vi "AlliGator Get Optimal IRF from Decay v2.vi"(8 "error in (no error)":errorcluster, 11 "Selected Plot Info":T2={"Multiplot XY Graph"=refnum, "Mouse Coordinates"={"Horizontal"=0, "Vertical"=0}, "Plot Index"=-1}) -> (0 "Error Out":errorcluster, 2 "Message":string, 3 "Extracted IRF":cluster{"t Array":dbl[], "IRF Array":dbl[]})   [LabVIEW 2021, in "AlliGator IRF.lvlib"]
doc: "Extract IRF from single-exponential decay by deconvolution and optimization of the time constant."
uses:
  AlliGator IRF.lvlib
  Graphs/XY Graph/XY Graph Selected Plot Info.ctl
  Graphs/XY Graph/XY Graph Refnum.ctl
  <vilib>/Utility/miscctls.llb/LVPoint32TypeDef.ctl
  Settings/AlliGator Settings List.ctl
  AlliGator IRF Optimization Controls.ctl
  AlliGator IRF Deconvolution Metrics.ctl
  Fits/IRF(X)PSED/IRF(X)PSED Fixed Parameters v3.ctl
  Fits/IRF(X)PSED/IRF(X)PSED Extraction Options.ctl
  Fits/IRF(X)PSED/Fourier Series Smoothing Option.ctl
  Fits/IRF(X)PSED/Fourier Series Truncation.ctl
  Fits/IRF(X)PSED/IRF Extraction Method.ctl
  Fits/IRF(X)PSED/Decay Fit Options v4.ctl
  Fits/Decay Convolution/Decay Model.ctl
  Fits/Residual Type.ctl
  Fits/IRF(X)PSED/Fit Weights Type v2.ctl
  Fits/Non-linear Fitting Method v2.ctl
  Fits/Fit Calculation Method.ctl
  Fits/Non-linear Fitting Algorithm.ctl
  Variant/Variant to Data/Variant to I32.vi
  Graphs/XY Graph/XY Graph Add Single Plot with Name.vi
  Graphs/XY Graph/XY Graph Add-Ons.lvlib
  Settings/AlliGator Settings.lvlib
  Notebook/Notebook.lvlib
  Fits/Fits.lvlib
  Variant/Variant to Data/Variant to Data.lvlib
panel:
  in  "Tab Control":T1(tab)
  out "Optimization Graph":cluster{"X Array":dbl[], "Y Array":dbl[]}[](graph)
  out "Power Spectrum Graph":dbl[][](graph)
  in  "Plot Names":string[](array[string])=["Tail Average", "Tail Average SG", "Tail SDV", "Tail SDV S-G", "Tail Max", "Tail Max S-G", "Tail SDV x Average", "Tail SDV x Average S-G", "Slope", "Slope S-G", "Residuals ACF SDV", "Residuals ACF SDV S-G", "Delta tau", "Delta tau S-G"]
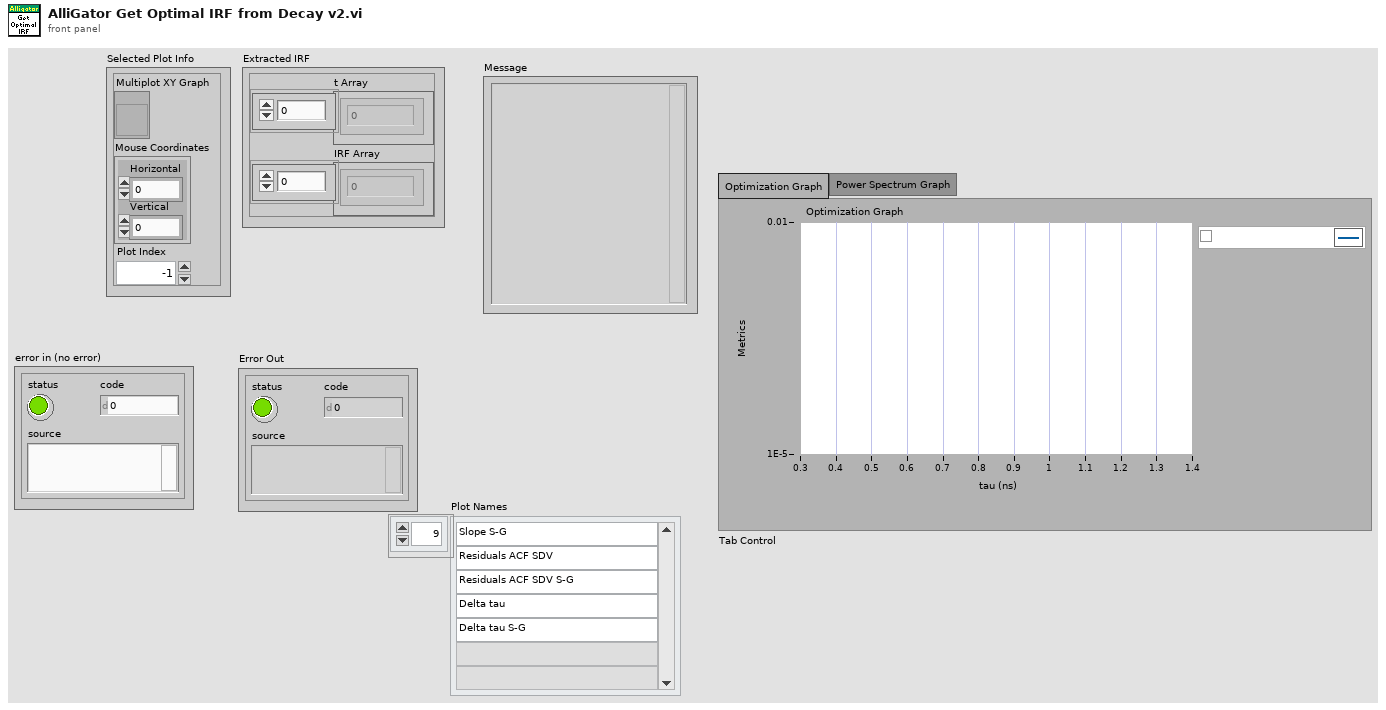
[diagram p1: front panel]
types:
  T1 = enum32{"Optimization Graph", "Power Spectrum Graph"}
  T2 = typedef "XY Graph Add-Ons.lvlib/XY Graph Selected Plot Info.ctl" = cluster{"Multiplot XY Graph":T3, "Mouse Coordinates":T4, "Plot Index":i32}
  T3 = typedef "XY Graph Add-Ons.lvlib/XY Graph Refnum.ctl" = refnum<vi>
  T4 = typedef "LVPoint32TypeDef.ctl" = cluster{"Horizontal":i32, "Vertical":i32}
  T5 = typedef "Fits.lvlib/IRF(X)PSED Extraction Options.ctl" = cluster{"Time Constant for IRF Extraction":dbl[unit], "IRF Order":i32, "Fourier Series Smoothing":T6, "Noise Threshold":dbl, "Smoothing Width":dbl, "Fourier Series Truncation":T7, "Truncation Order":i32, "Save Power Spectrum":bool, "Smoothing":bool, "Smoothing Parameter":dbl, "Smoothing Order":u32, "Method":T8}
  T6 = typedef "Fits.lvlib/Fourier Series Smoothing Option.ctl" = enum16{"None", "Lanczos Factors", "Fejer Summation"}
  T7 = typedef "Fits.lvlib/Fourier Series Truncation.ctl" = enum16{"Automatic", "Fixed"}
  T8 = typedef "Fits.lvlib/IRF Extraction Method.ctl" = enum16{"Direct", "Topless", "Toeplitz"}
  T9 = typedef "Fits.lvlib/IRF(X)PSED Fixed Parameters v3.ctl" = cluster{"order":i32, "T":dbl, "Time Constant Array":dbl[], "{S_k, C_k, phi_k, e_k} arrays":cluster{"S_k Array":dbl[], "C_k Array":dbl[], "phi_k Array":dbl[], "e_k Array":dbl[]}, "IRF Extraction Options":T5}
  T10 = typedef "AlliGator Settings.lvlib/AlliGator Settings List.ctl" = enum16{"GUI:Visible Settings Tab", "GUI:Last Run Version", "Source Image:Use Image Histogram for Contrast", "Source Image:Low Count Pixels Rejection Options", "Source Image:High Count Pixels Rejection Options", "Source Image:Use Image Brightness", "Source Image:Blend Overlay with Image Background", "Source Image:Use Fixed ROI Diameter", "Source Image:ROI Diameter", "Source Image:ROI Center Color", "Source Image:Peak Threshold", "Source Image:Intensity Threshold", "Source Image:Image Binning Options", "Source Image:Image Smoothing Options", "Source Image:Image Histogram Active", "Source Image:Invert Binary Mask", "Source Image:Hot Pixel Removal", "Source Image:Overlay Analyzed ROI Center", "Source Image:Auto-Adjust Contrast", "Source Image:Histogram Lower Percentile", "Source Image:Histogram Upper Percentile", "Source Image:Save Source Image", "Source Image:Scale Bar Options", "Source Image:Image Resolution (Pixel Size)", "Source Image:Flatfield Correction", "Source Image:Show Dead Left Columns Correction", "Source Image:Dead Left Columns Correction", "Source Image:Image Pre-Processing Operations Order", "Source Image:Overlay ROI Median", "Source Image:Median Overlay Color", "Data Information:Gate Width", "Data Information:Nanotime Gate Separation", "Data Information:Macrotime Gate Separation", "Data Information:Gate Step", "Data Information:# Gates", "Data Information:Gate Image Exposure", "Data Information:Gate Image Integration", "Data Information:Gates to Skip", "Data Information:Gates to Keep", "Data Information:Define Gates to", "Data Information:Channel Name", "Data Information:Available Channel Names", "Data Information:Channel Arithmetic", "Data Information:Background File Subtraction", "Data Information:Background File", "Data Information:Background Scaling Factor", "Data Information:Background Pile-up Correction", "Data Information:Background Pixel Well Capacity", "Data Information:Laser Period", "Data Information:SYNC Period", "Data Information:Pile-up Correction", "Data Information:Pixel Well Capacity", "Data Information:Dataset Scaling Factor", "Fluorescence Decay_Decay Pre-Processing:Reverse Gates", "Fluorescence Decay_Decay Pre-Processing:Verbose Decay Pre-Processing", "Fluorescence Decay_Decay Pre-Processing:Use Decay Pre-Processing", "Fluorescence Decay_Decay Pre-Processing:Background Subtraction", "Fluorescence Decay_Decay Pre-Processing:Background Definition Range", "Fluorescence Decay_Decay Pre-Processing:Baseline Subtraction Method", "Fluorescence Decay_Decay Pre-Processing:Decay Pre-Processing Operations Order", "Fluorescence Decay_Decay Pre-Processing:Smoothing Parameter", "Fluorescence Decay_Decay Pre-Processing:Shift Decay", "Fluorescence Decay_Decay Pre-Processing:Decay Shift Parameters", "Fluorescence Decay_Decay Pre-Processing:Fold Decay", "Fluorescence Decay_Decay Pre-Processing:# Folds", "Fluorescence Decay_Decay Pre-Processing:1-Normalize Decay", "Fluorescence Decay_Decay Pre-Processing:[0-1]-Normalize Decay", "Fluorescence Decay_Decay Pre-Processing:Smoothen Decay", "Fluorescence Decay_Decay Pre-Processing:Extrapolate Decay", "Fluorescence Decay_Decay Pre-Processing:Use Periodicity", "Fluorescence Decay_Decay Pre-Processing:Use Cursors", "Fluorescence Decay_Decay Pre-Processing:Tail Fraction", "Fluorescence Decay_Decay Pre-Processing:Head Fraction", "Fluorescence Decay_Decay Pre-Processing:Additional Points", "Fluorescence Decay_Decay Pre-Processing:Straighten Decay", "Fluorescence Decay_Decay Pre-Processing:Constant Background", "Fluorescence Decay_Decay Pre-Processing:Pixel-Normalize Decay", "Fluorescence Decay_Advanced Analysis:Extract IRF instead of Decay", "Fluorescence Decay_Advanced Analysis:IRF Extraction Options", "Fluorescence Decay_Advanced Analysis:IRF Optimization Options", "Fluorescence Decay_Advanced Analysis:Square Pulse Options", "Fluorescence Decay_Advanced Analysis:IRF Order", "Fluorescence Decay_Advanced Analysis:IRF Time Constants", "Fluorescence Decay_Advanced Analysis:Wavelet Analysis Options", "Fluorescence Decay_Advanced Analysis:Average Lifetime Options", "Fluorescence Decay_Fit Options:Fit Options", "Fluorescence Decay_Fit Options:Use Legacy Fitting Approach", "Fluorescence Decay_Fit Options:Use Data Information Laser Period", "Fluorescence Decay_Fit Parameters:Displayed Fit Parameters", "Fluorescence Decay_Fit Parameters:Fit Parameter Constraints", "Fluorescence Decay_Fit Parameters:Export Tabulated Results", "Fluorescence Decay_Fit Parameters:MLE Baseline Offset Type", "Fluorescence Decay_Fit Parameters:MLE Baseline Offset", "Fluorescence Decay_Fit Parameters:Guess Parameter Names", "Fluorescence Decay_Fit Parameters:Guess Parameter Values", "Fluorescence Decay_Fit Parameters:Guess Parameters Options", "Fluorescence Decay_Fit Parameters:Optimal Offset Selection Criterion", "Fluorescence Decay_Styles:Show Last Decay Only", "Fluorescence Decay_Styles:Decay Graph Color Array", "Fluorescence Decay:Decay Graph Active", "Fluorescence Decay Statistics:Min Peak Value", "Fluorescence Decay Statistics:Reject Low Decay Peak Pixels", "Fluorescence Decay Statistics:Reject High Decay Peak Pixels", "Fluorescence Decay Statistics:Max Peak Value", "Time Traces:Use File Timestamp", "Time Traces:Time Step", "Time Traces:Use Intensity Correction File", "Time Traces:Intensity Correction File", "Phasor Plot:Phasor Plot Smoothing Options", "Phasor Plot:Phasor Plot Size", "Phasor Plot:Phasor Plot Graphics Options", "Phasor Plot:Cumulative Phasor Plot", "Phasor Plot:Use Phasor Brightness", "Phasor Plot:Blend Overlay with Phasor Background", "Phasor Plot:Save Phasor Plot", "Phasor Plot:Show References", "Phasor Plot:Phasor Ratio Decay Range", "Phasor Plot:Exponential Fading", "Phasor Plot:Phasor Ratio Reference Colors", "Phasor Plot:Reference Radius", "Phasor Plot:Show Color Map Vertices", "Phasor Plot:Phasor Plot Active", "Phasor Plot:Phasor Ratio Color Map Type", "Phasor Plot:Phasor Ratio Color Map", "Phasor Plot:Phasor Ratio Display Range", "Phasor Plot:Selected Image ROI(s)", "Phasor Plot:All Image ROIs", "Phasor Plot:Selected Phasor Plot ROI(s)", "Phasor Plot:All Phasor Plot ROIs", "Phasor Plot:Phasor Ratio Color-Coded Quantity", "Phasor Plot:Store Phasor Harmonics", "Phasor Plot:Draw Reference Segment", "Phasor Plot:User-Defined Quantity", "Phasor Plot:Color Scale High Color", "Phasor Plot:Color Scale Low Color", "Phasor Plot:Intensity-weighted Phasor Plot", "Phasor Graph:Phasor Frequency", "Phasor Graph:Phasor Ratio Type", "Phasor Graph:Pixel-level Phasor Computation", "Phasor Graph:Save Phasor Graph", "Phasor Graph:Phasor Graph Active", "Phasor Graph:Phasor SDV Options", "Phasor Graph:Intensity-weighted Phasor Graph", "Phasor Graph:Define Shortest Lifetime as", "Phasor Calibration:Use Backup Calibration if needed", "Phasor Calibration:Backup Calibration Type", "Phasor Calibration:Calibration Type", "Phasor Calibration:Calibration Lifetime", "Phasor Calibration:Calibration Map Algorithm", "Single-Exponential Phasor Locus (SEPL):Gate Parameters", "Single-Exponential Phasor Locus (SEPL):User-defined Gate", "Single-Exponential Phasor Locus (SEPL):User-defined IRF", "Single-Exponential Phasor Locus (SEPL):Phasor Parameters", "Single-Exponential Phasor Locus (SEPL):Decay & IRF Parameters", "Single-Exponential Phasor Locus (SEPL):Display Parameters", "Lifetime Analysis:Decay Analysis Parameters", "Lifetime Analysis:Lifetime Map Active", "Plugins:Python Settings", "Miscellaneous:Verbose Mode", "Miscellaneous:Beep after Script", "Miscellaneous:Saved Image File Format", "Miscellaneous:Exported Gate Image Settings", "Miscellaneous:Include Loading in Timing", "Miscellaneous:Verbose Settings Mode", "Miscellaneous:Histogram Options", "Miscellaneous:Beep on Error", "Miscellaneous:# Logical Processors Used", "Miscellaneous:ROI Description Max Characters", "Miscellaneous:Verbose Error Mode", "Miscellaneous:Transparent Mask Color"}
  T11 = typedef "AlliGator IRF.lvlib/AlliGator IRF Optimization Controls.ctl" = cluster{"Search Range":dbl[unit], "Search Step":dbl[unit], "Tail Threshold (%)":dbl, "Regularized IRF":bool, "Export Plot":bool, "Export Data":bool, "Smooth Metrics":bool, "S-G Side Points":i32, "S-G Polynomial Order":i32, "Metrics":T12}
  T12 = typedef "AlliGator IRF.lvlib/AlliGator IRF Deconvolution Metrics.ctl" = enum16{"Average", "SDV", "Max", "Average * SDV", "Slope", "Residual ACF SDV", "Delta tau", "Reduced Chi2"}
  T13 = typedef "Fits.lvlib/Decay Fit Options v4.ctl" = cluster{"Show Fit Residuals":bool, "Fit Model":T14, "Residual Type":T15, "Max Decay Percentile":dbl, "Min Decay Percentile":dbl, "Show Full Decay":bool, "Weights":T16, "Fitting Method":T17, "Compute Parameter Uncertainties":bool, "Periodic Boundaries":bool, "Model Calculation":T18, "Period":dbl[unit], "Termination Criteria":cluster{"Max Iterations":i32, "Max Function Calls":i32, "Max Time":dbl[unit], "Function Tolerance":dbl, "Parameter Tolerance":dbl, "Gradient Tolerance":dbl, "Min Lambda":dbl, "Max Lambda":dbl, "Initial Tick Count":u32}, "Offset Resolution":dbl[unit], "Use Local IRF":bool, "Fitting Algorithm":T19, "Show Confidence Interval ":bool, "Confidence Level":dbl}
  T14 = typedef "Fits.lvlib/Decay Model.ctl" = enum16{"1-Exponential", "2-Exponentials"}
  T15 = typedef "Fits.lvlib/Residual Type.ctl" = enum16{"Standard", "Normalized", "Reduced"}
  T16 = typedef "Fits.lvlib/Fit Weights Type v2.ctl" = enum16{"Unweighted", "1/Variance (Neyman)", "1/Variance (Pearson)", "Best of All"}
  T17 = typedef "Fits.lvlib/Non-linear Fitting Method v2.ctl" = enum16{"Least Square", "Least Absolute Residual", "Bisquare", "MLE", "-", "Best of All"}
  T18 = typedef "Fits.lvlib/Fit Calculation Method.ctl" = enum16{"Simulation", "Convolution", "Integration"}
  T19 = typedef "Fits.lvlib/Non-linear Fitting Algorithm.ctl" = enum16{"Levenberg-Marquardt", "Trust-Region Dogleg"}
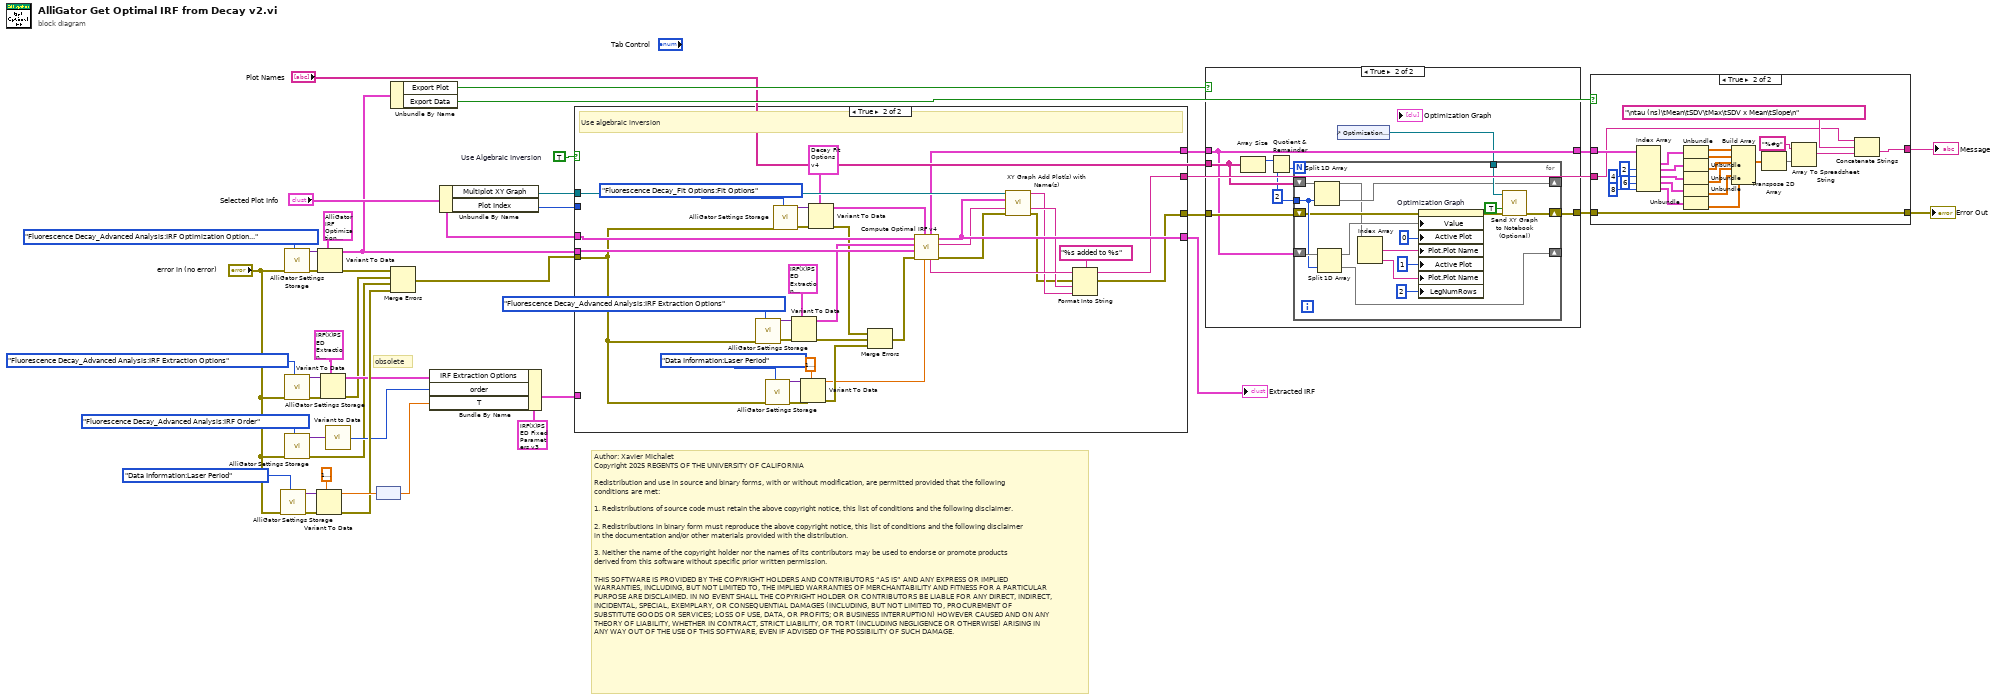
[diagram p0: block diagram]
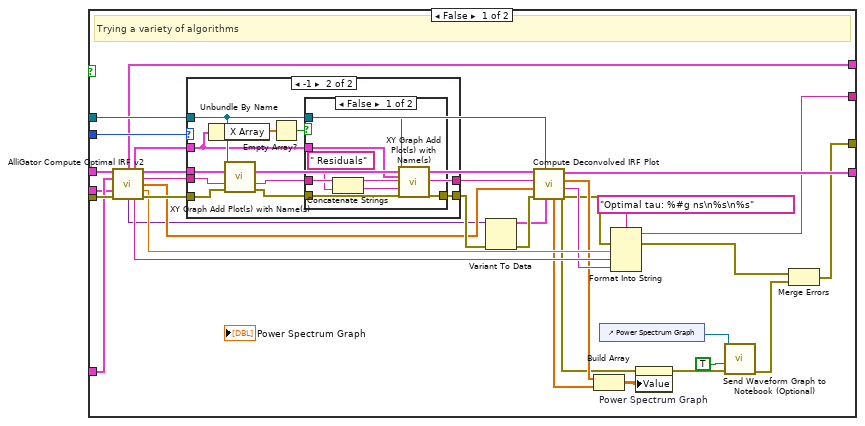
[diagram p4: hidden frame]
diagram:
  w12 = TRUE  # Use Algebraic Inversion
  # "Author: Xavier Michalet\nCopyright 2025 REGENTS OF THE UNIVERSITY OF CALIFORNIA\n\nRedistribution and use in source and binary forms, with or without modification, are permitted provided that the following conditions are met:\n\n1. Redistributions of source code must retain the above copyright notice, this list of conditions and the following disclaimer.\n\n2. Redistributions in binary form must reproduce the above copyright notice, this list of conditions and the following disclaimer in the documentation and/or other materials provided with the distribution.\n\n3. Neither the name of the copyright holder nor the names of its contributors may be used to endorse or promote products derived from this software without specific prior written permission.\n\nTHIS SOFTWARE IS PROVIDED BY THE COPYRIGHT HOLDERS AND CONTRIBUTORS “AS IS” AND ANY EXPRESS OR IMPLIED WARRANTIES, INCLUDING, BUT NOT LIMITED TO, THE IMPLIED WARRANTIES OF MERCHANTABILITY AND FITNESS FOR A PARTICULAR PURPOSE ARE DISCLAIMED. IN NO EVENT SHALL THE COPYRIGHT HOLDER OR CONTRIBUTORS BE LIABLE FOR ANY DIRECT, INDIRECT, INCIDENTAL, SPECIAL, EXEMPLARY, OR CONSEQUENTIAL DAMAGES (INCLUDING, BUT NOT LIMITED TO, PROCUREMENT OF SUBSTITUTE GOODS OR SERVICES; LOSS OF USE, DATA, OR PROFITS; OR BUSINESS INTERRUPTION) HOWEVER CAUSED AND ON ANY THEORY OF LIABILITY, WHETHER IN CONTRACT, STRICT LIABILITY, OR TORT (INCLUDING NEGLIGENCE OR OTHERWISE) ARISING IN ANY WAY OUT OF THE USE OF THIS SOFTWARE, EVEN IF ADVISED OF THE POSSIBILITY OF SUCH DAMAGE."
  # "obsolete"
  n1 = call "AlliGator Settings Storage.vi"("AlliGator Settings List"=AlliGator_Settings_List."Data Information:Laser Period", "Error In"="error in (no error)") -> ("Error Out"=w32:errorcluster, "Variant Data out"=w34:variant)  [unwired: 8 in]
  n2 = call "AlliGator Settings Storage.vi"("AlliGator Settings List"=AlliGator_Settings_List."Fluorescence Decay_Advanced Analysis:IRF Optimization Options", "Error In"="error in (no error)") -> ("Error Out"=w40:errorcluster, "Variant Data out"=w41:variant)  [unwired: 8 in]
  n3 = call "AlliGator Settings Storage.vi"("AlliGator Settings List"=AlliGator_Settings_List."Fluorescence Decay_Advanced Analysis:IRF Extraction Options", "Error In"="error in (no error)") -> ("Error Out"=w26:errorcluster, "Variant Data out"=w27:variant)  [unwired: 8 in]
  n4 = call "AlliGator Settings Storage.vi"("AlliGator Settings List"=AlliGator_Settings_List."Fluorescence Decay_Advanced Analysis:IRF Order", "Error In"="error in (no error)") -> ("Error Out"=w19:errorcluster, "Variant Data out"=w25:variant)  [unwired: 8 in]
  n5 = Variant To Data(error in=w32, type=dbl[unit] 1e-09 ("Time Constant"), Variant=w34) -> (data=w31:dbl[unit], error out=w29:errorcluster)
  n6 = Variant To Data(error in=w40, type=T11 {"Search Range"=1e-09, "Search Step"=1e-09, "Tail Threshold (%)"=1.0, "Regularized IRF"=FALSE, "Export Plot"=FALSE, "Export Data"=FALSE, "Smooth Metrics"=FALSE, "S-G Side Points"=1, "S-G Polynomial Order"=3, "Metrics"=enum."Average"} ("IRF Optimization Control"), Variant=w41) -> (data=w11:T11, error out=w37:errorcluster)
  n7 = Variant To Data(error in=w26, type=T5 {"Time Constant for IRF Extraction"=4.08e-09, "IRF Order"=132, "Fourier Series Smoothing"=enum."Fejer Summation", "Noise Threshold"=0.1, "Smoothing Width"=0.1, "Fourier Series Truncation"=enum."Automatic", "Truncation Order"=0, "Save Power Spectrum"=FALSE, "Smoothing"=FALSE, "Smoothing Parameter"=0.0, "Smoothing Order"=1, "Method"=enum."Direct"} ("IRF Extraction Options"), Variant=w27) -> (data=w22:T5, error out=w20:errorcluster)
  n8 = call-poly "Variant to Data.vi"("Variant"=w25) -> ("Value"=w21:i32)  [unwired: 8 in]
  n9 = node(w31) -> (w18:dbl)
  n10 = Unbundle By Name(w11) -> ("Export Plot"=w8:bool, "Export Data"=w7:bool)
  n11 = Merge Errors(w37, w20, w19, w29) -> (w30:errorcluster)
  n12 = Bundle By Name(cluster=T9 {"order"=0, "T"=0.0, "Time Constant Array"=[], "{S_k, C_k, phi_k, e_k} arrays"={"S_k Array"=[], "C_k Array"=[], "phi_k Array"=[], "e_k Array"=[]}, "IRF Extraction Options"={"Time Constant for IRF Extraction"=1e-18, "IRF Order"=0, "Fourier Series Smoothing"=enum."None", "Noise Threshold"=0.0, "Smoothing Width"=0.0, "Fourier Series Truncation"=enum."Automatic", "Truncation Order"=0, "Save Power Spectrum"=FALSE, "Smoothing"=FALSE, "Smoothing Parameter"=0.0, "Smoothing Order"=1, "Method"=enum."Direct"}} ("IRF*PSED Fixed Parameters"), "IRF Extraction Options"=w22, "order"=w21, "T"=w18) -> (w14:T9)
  n13 = Unbundle By Name("Selected Plot Info") -> ("Multiplot XY Graph"=w15:T3, "Plot Index"=w16:i32)
  n14 = case shown="True" w12 {
    tunnel: "Selected Plot Info" -> [w74 w129]
    tunnel: [w73 w127] -> w36
    tunnel: w30 -> [w72 w98]
    tunnel: w16 -> [w71 _]
    tunnel: w15 -> [w70 w128]
    tunnel: [w65 w119] -> w9
    tunnel: w14 -> [w61 _]
    tunnel: w11 -> [w45 w118]
    tunnel: [w44 w117] -> w10
    tunnel: [w43 w116] -> w3
    frame False {
      # "Trying a variety of algorithms"
      n15 = call "AlliGator Compute Optimal IRF v2.vi"("Selected Plot Info"=w74, "IRF*PSED Fixed Parameters"=w61, "IRF Optimization Control"=w45, "Error In"=w72) -> ("Optimization Graph"=w44:cluster{"Ramp Pattern":dbl[], dbl[]}[], "Residuals Plot"=w64:cluster{"X Array":dbl[], "Y Array":dbl[]}, "Fitted Plot"=w69:cluster{"X Array":dbl[], "Y Array":dbl[]}, "Plot Name"=w68:string, "Fit Parameter Values"=w56:dbl[], "Optimal Tau"=w62:dbl, "Additional Data"=w55:variant, "Fit Results String"=w63:string, "Error Out"=w67:errorcluster)  [unwired: 3 in]
      n16 = case shown="-1" w71 {
        tunnel: w70 -> [_ w80]
        tunnel: w69 -> [_ w87]
        tunnel: w68 -> [w77 w86]
        tunnel: w67 -> [w76 w85]
        tunnel: [w77 w78] -> w66
        tunnel: [w76 w81] -> w60
        tunnel: w64 -> [_ w79]
        frame 0, Default {
          # "if programmatic do not plot the fit\nbut the IRF  only"
        }
        frame -1 {
          n17 = Unbundle By Name(w79) -> ("X Array"=w84:dbl[])
          n18 = call-poly "XY Graph Add Plot(s) with Name(s).vi"("XYGraph Ref in"=w80, "Plot"=w87, "Plot Name (\"Plot\")"=w86, "error in (no error)"=w85) -> ("Plot Name"=w78:string, "error out"=w82:errorcluster)  [unwired: 8 in, 2 out]
          n19 = Empty Array?(array=w84) -> (empty?=w83:bool)
          n20 = case shown="False" w83 {
            tunnel: w82 -> [w94 w95]
            tunnel: [w93 w95] -> w81
            tunnel: w80 -> [w92 _]
            tunnel: w79 -> [w91 _]
            tunnel: w78 -> [w90 _]
            frame False {
              n21 = Concatenate Strings(w90, " Residuals" ("string")) -> (w88:string)
              n22 = call-poly "XY Graph Add Plot(s) with Name(s).vi"("XYGraph Ref in"=w92, "Plot"=w91, "Plot Name (\"Plot\")"=w88, "error in (no error)"=w94) -> ("error out"=w93:errorcluster)  [unwired: 8 in, 3 out]
            }
            frame True {
            }
          }
        }
      }
      n23 = Variant To Data(error in=w60, Variant=w55) -> (data=w58:T9, error out=w59:errorcluster)  [unwired: 1 in]
      n24 = call "Compute Deconvolved IRF Plot.vi"("IRF*PSED fixed Parameters"=w58, "XYGraph in"=w70, "error in (no error)"=w59, "Fit Parameter Values"=w56, "Plot Name"=w66, "Fitted Decay"=w69) -> ("error out"=w53:errorcluster, "Amplitude String"=w57:string, "Power Spectrum"=w54:dbl[], "IRF Plot"=w73:cluster{"X Array":dbl[], "Y Array":dbl[]}, "Smoothed Power Spectrum"=w48:dbl[])  [unwired: 1 in]
      n25 = Build Array(w54, w48) -> (w46:dbl[][])
      n26 = control-ref of="Power Spectrum Graph"() -> (w50:refnum<vi>)
      n27 = Format Into String(format string="Optimal tau: %#g ns\n%s\n%s", error in=w53, w62, w63, w57) -> (resulting string=w43:string, error out=w47:errorcluster)  [unwired: 1 in]
      n28 = property on="Power Spectrum Graph" class="WFGraph (strict)"(error in=w53, "Value"=w46) -> (error out=w52:errorcluster)  [unwired: 1 in, 1 out]
      n29 = call "Send Waveform Graph to Notebook (Optional).vi"("error in (no error)"=w52, "Send Graph to Notebook?"=TRUE, "Multiwaveform Graph Refnum"=w50) -> ("error out"=w49:errorcluster)  [unwired: 8 in]
      n30 = Merge Errors(w47, w49) -> (w65:errorcluster)
    }
    frame True {
      # "Use algebraic inversion"
      n31 = call "AlliGator Settings Storage.vi"("AlliGator Settings List"=AlliGator_Settings_List."Fluorescence Decay_Advanced Analysis:IRF Extraction Options", "Error In"=w98) -> ("Error Out"=w113:errorcluster, "Variant Data out"=w115:variant)  [unwired: 8 in]
      n32 = call "AlliGator Settings Storage.vi"("AlliGator Settings List"=AlliGator_Settings_List."Data Information:Laser Period", "Error In"=w98) -> ("Error Out"=w108:errorcluster, "Variant Data out"=w109:variant)  [unwired: 8 in]
      n33 = call "AlliGator Settings Storage.vi"("AlliGator Settings List"=AlliGator_Settings_List."Fluorescence Decay_Fit Options:Fit Options", "Error In"=w98) -> ("Error Out"=w102:errorcluster, "Variant Data out"=w101:variant)  [unwired: 8 in]
      n34 = Variant To Data(error in=w113, type=T5 {"Time Constant for IRF Extraction"=1e-18, "IRF Order"=1, "Fourier Series Smoothing"=enum."None", "Noise Threshold"=0.0, "Smoothing Width"=0.0, "Fourier Series Truncation"=enum."Automatic", "Truncation Order"=0, "Save Power Spectrum"=FALSE, "Smoothing"=FALSE, "Smoothing Parameter"=0.0, "Smoothing Order"=1, "Method"=enum."Direct"} ("IRF Extraction Options"), Variant=w115) -> (data=w104:T5, error out=w112:errorcluster)
      n35 = Variant To Data(error in=w108, type=dbl[unit] 1e-09 ("Time Constant"), Variant=w109) -> (data=w103:dbl[unit], error out=w105:errorcluster)
      n36 = Variant To Data(error in=w102, type=T13 {"Show Fit Residuals"=TRUE, "Fit Model"=enum."1-Exponential", "Residual Type"=enum."Standard", "Max Decay Percentile"=0.0, "Min Decay Percentile"=0.0, "Show Full Decay"=TRUE, "Weights"=enum."Unweighted", "Fitting Method"=enum."Least Square", "Compute Parameter Uncertainties"=TRUE, "Periodic Boundaries"=TRUE, "Model Calculation"=enum."Simulation", "Period"=1.2500000000000001e-08, "Termination Criteria"={"Max Iterations"=0, "Max Function Calls"=0, "Max Time"=1000.0, "Function Tolerance"=1e-06, "Parameter Tolerance"=1e-06, "Gradient Tolerance"=0.0, "Min Lambda"=1e-06, "Max Lambda"=1e-06, "Initial Tick Count"=0}, "Offset Resolution"=1.2500000000000001e-08, "Use Local IRF"=TRUE, "Fitting Algorithm"=enum."Levenberg-Marquardt", "Show Confidence Interval "=TRUE, "Confidence Level"=95.0} ("Decay Fit Options"), Variant=w101) -> (data=w96:T13, error out=w97:errorcluster)
      n37 = Merge Errors(w97, w112, w105) -> (w111:errorcluster)
      n38 = call "Compute Optimal IRF v4.vi"("Laser Period"=w103, "Decay Fit Options"=w96, "Error In"=w111, "IRF Optimization Control"=w118, "Extract IRF Options"=w104, "Selected Plot Info"=w129) -> ("Error Out"=w125:errorcluster, "Plot Name"=w126:string, "IRF Plot"=w127:cluster{"X Array":dbl[], "Y Array":dbl[]}, "Optimal IRF Results String"=w124:string, "Optimization Graph"=w117:cluster{dbl[], dbl[]}[])  [unwired: 1 out]
      n39 = call-poly "XY Graph Add Plot(s) with Name(s).vi"("XYGraph Ref in"=w128, "Plot"=w127, "Plot Name (\"Plot\")"=w126, "error in (no error)"=w125) -> ("XY Graph Caption (or Label)"=w121:string, "Plot Name"=w123:string, "error out"=w120:errorcluster)  [unwired: 8 in, 1 out]
      n40 = Format Into String(format string="%s added to %s", initial string=w124, error in=w120, w123, w121) -> (resulting string=w116:string, error out=w119:errorcluster)
    }
  }
  "Extracted IRF" <- w36
  n41 = case shown="True" w8 {
    tunnel: w10 -> [w130 w134]
    tunnel: w9 -> [w131 w139]
    tunnel: [w131 w132] -> w6
    tunnel: [w130 w134] -> w4
    tunnel: "Plot Names" -> [_ w136]
    frame False {
    }
    frame True {
      w135 = 2 ("y")
      n42 = Array Size(array=w136) -> (size(s)=w138:i32)
      n43 = Quotient & Remainder(x=w138, y=w135) -> (floor(x/y)=w137:i32)  [unwired: 1 out]
      n44 = control-ref of="Optimization Graph"() -> (w133:refnum<vi>)
      n45 = for {
        N: w137 -> [_]
        tunnel: w133 -> [w155]
        shift-right: [w154] -> w132
        shift-left: w139 -> [w149]
        shift-right: [w152] -> _
        shift-left: w136 -> [w153]
        tunnel: w135 -> [w150]
        shift-right: [w145] -> _
        shift-left: w134 -> [w151]
        n46 = Split 1D Array(array=w153, index=w150) -> (first subarray=w143:string[], second subarray=w152:string[])
        n47 = Split 1D Array(array=w151, index=w150) -> (first subarray=w147:cluster{"Ramp Pattern":dbl[], dbl[]}[], second subarray=w145:cluster{"Ramp Pattern":dbl[], dbl[]}[])
        n48 = Index Array(array=w143) -> (element #1=w142:string, element #2=w141:string)  [unwired: 2 in]
        n49 = property on="Optimization Graph" class="XYGraph (strict)"(error in=w149, "Value"=w147, "Active Plot"=u32 0, "Plot.Plot Name"=w142, "Active Plot"=u32 1, "Plot.Plot Name"=w141, "LegNumRows"=u32 2 ("Legend:Number of Rows")) -> (error out=w148:errorcluster)  [unwired: 1 in, 1 out]
        n50 = call "Send XY Graph to Notebook (Optional).vi"("error in (no error)"=w148, "Send Graph to Notebook?"=TRUE, "XYGraph in"=w155) -> ("error out"=w154:errorcluster)  [unwired: 8 in]
      }
    }
  }
  n51 = case shown="True" w7 {
    tunnel: w6 -> [w158 w175]
    tunnel: [w158 w175] -> w5
    tunnel: w4 -> [_ w182]
    tunnel: w3 -> [w157 w165]
    tunnel: [w157 w166] -> w2
    frame False {
    }
    frame True {
      n52 = Index Array(array=w182, index #2=2 ("index"), index #3=4 ("index"), index #4=6 ("index"), index #5=8 ("index")) -> (element #1=w181:cluster{"Ramp Pattern":dbl[], dbl[]}, element #2=w173:cluster{"Ramp Pattern":dbl[], dbl[]}, element #3=w172:cluster{"Ramp Pattern":dbl[], dbl[]}, element #4=w168:cluster{"Ramp Pattern":dbl[], dbl[]}, element #5=w161:cluster{"Ramp Pattern":dbl[], dbl[]})  [unwired: 1 in]
      n53 = Unbundle(w181) -> ("Ramp Pattern"=w180:dbl[], w179:dbl[])
      n54 = Unbundle(w173) -> (w171:dbl[])  [unwired: 1 out]
      n55 = Unbundle(w172) -> (w170:dbl[])  [unwired: 1 out]
      n56 = Unbundle(w168) -> (w167:dbl[])  [unwired: 1 out]
      n57 = Unbundle(w161) -> (w159:dbl[])  [unwired: 1 out]
      n58 = Build Array(w180, w179, w171, w170, w167, w159) -> (w178:dbl[][])
      n59 = Transpose 2D Array(2D array=w178) -> (transposed array=w174:dbl[][])
      n60 = Array To Spreadsheet String(array=w174, 3:"%#g" ("format string")) -> (spreadsheet string=w176:string)  [unwired: 1 in]
      n61 = Concatenate Strings(w165, "\ntau (ns)\tMean\tSDV\tMax\tSDV x Mean\tSlope\n" ("string"), w176) -> (w166:string)
    }
  }
  "Error Out" <- w5
  "Message" <- w2
